vi "Dialog_TestGIV (SubVI).vi"() -> ()   [LabVIEW 2017]
uses:
  <vilib>/Waveform/WDTFileIO.llb/ Write Waveforms to File (1D).vi
panel:
  in  "Stop":bool
  in  "ExpClipboard":bool
  in  "UNDT_NOut":u8=1 caption="№ ПЭП подкл. к ГИВ" min=1 max=8 step=1
  out "Horizontal Fill Indicator":dbl(slide)=1.0 scale=0.0..1.0
  in  "Tab Control 2":enum32{"Osc", "Table", "Parameters"}(tab)
  out "OscPulse":waveform(dbl)[](graph)=[{"t0"=timestamp(0 s since 1904-01-01), "dt"=2.000000026702864e-10, "Y"=array[2502 elements]}, {"t0"=timestamp(0 s since 1904-01-01), "dt"=2.000000026702864e-10, "Y"=array[2502 elements]}, {"t0"=timestamp(0 s since 1904-01-01), "dt"=2.000000026702864e-10, "Y"=array[2502 elements]}, {"t0"=timestamp(0 s since 1904-01-01), "dt"=2.000000026702864e-10, "Y"=array[2502 elements]}, {"t0"=timestamp(0 s since 1904-01-01), "dt"=2.000000026702864e-10, "Y"=array[2502 elements]}, {"t0"=timestamp(0 s since 1904-01-01), "dt"=2.000000026702864e-10, "Y"=array[2502 elements]}, {"t0"=timestamp(0 s since 1904-01-01), "dt"=4.000000053405728e-10, "Y"=array[5002 elements]}, {"t0"=timestamp(0 s since 1904-01-01), "dt"=4.000000053405728e-10, "Y"=array[5002 elements]}, {"t0"=timestamp(0 s since 1904-01-01), "dt"=4.000000053405728e-10, "Y"=array[5002 elements]}, {"t0"=timestamp(0 s since 1904-01-01), "dt"=4.000000053405728e-10, "Y"=array[5002 elements]}, {"t0"=timestamp(0 s since 1904-01-01), "dt"=2.000000026702864e-10, "Y"=array[2502 elements]}, {"t0"=timestamp(0 s since 1904-01-01), "dt"=2.000000026702864e-10, "Y"=array[2502 elements]}, {"t0"=timestamp(0 s since 1904-01-01), "dt"=2.000000026702864e-10, "Y"=array[2502 elements]}, {"t0"=timestamp(0 s since 1904-01-01), "dt"=2.000000026702864e-10, "Y"=array[2502 elements]}, {"t0"=timestamp(0 s since 1904-01-01), "dt"=2.000000026702864e-10, "Y"=array[2502 elements]}, {"t0"=timestamp(0 s since 1904-01-01), "dt"=2.000000026702864e-10, "Y"=array[2502 elements]}, {"t0"=timestamp(0 s since 1904-01-01), "dt"=4.000000053405728e-10, "Y"=array[5002 elements]}, {"t0"=timestamp(0 s since 1904-01-01), "dt"=4.000000053405728e-10, "Y"=array[5002 elements]}, {"t0"=timestamp(0 s since 1904-01-01), "dt"=4.000000053405728e-10, "Y"=array[5002 elements]}, {"t0"=timestamp(0 s since 1904-01-01), "dt"=4.000000053405728e-10, "Y"=array[5002 elements]}, {"t0"=timestamp(0 s since 1904-01-01), "dt"=2.000000026702864e-10, "Y"=array[2502 elements]}, {"t0"=timestamp(0 s since 1904-01-01), "dt"=2.000000026702864e-10, "Y"=array[2502 elements]}, {"t0"=timestamp(0 s since 1904-01-01), "dt"=2.000000026702864e-10, "Y"=array[2502 elements]}, {"t0"=timestamp(0 s since 1904-01-01), "dt"=2.000000026702864e-10, "Y"=array[2502 elements]}, {"t0"=timestamp(0 s since 1904-01-01), "dt"=2.000000026702864e-10, "Y"=array[2502 elements]}, {"t0"=timestamp(0 s since 1904-01-01), "dt"=2.000000026702864e-10, "Y"=array[2502 elements]}, {"t0"=timestamp(0 s since 1904-01-01), "dt"=4.000000053405728e-10, "Y"=array[5002 elements]}, {"t0"=timestamp(0 s since 1904-01-01), "dt"=4.000000053405728e-10, "Y"=array[5002 elements]}, {"t0"=timestamp(0 s since 1904-01-01), "dt"=4.000000053405728e-10, "Y"=array[5002 elements]}, {"t0"=timestamp(0 s since 1904-01-01), "dt"=4.000000053405728e-10, "Y"=array[5002 elements]}, {"t0"=timestamp(0 s since 1904-01-01), "dt"=2.000000026702864e-10, "Y"=array[2502 elements]}, {"t0"=timestamp(0 s since 1904-01-01), "dt"=2.000000026702864e-10, "Y"=array[2502 elements]}, {"t0"=timestamp(0 s since 1904-01-01), "dt"=2.000000026702864e-10, "Y"=array[2502 elements]}, {"t0"=timestamp(0 s since 1904-01-01), "dt"=2.000000026702864e-10, "Y"=array[2502 elements]}, {"t0"=timestamp(0 s since 1904-01-01), "dt"=2.000000026702864e-10, "Y"=array[2502 elements]}, {"t0"=timestamp(0 s since 1904-01-01), "dt"=2.000000026702864e-10, "Y"=array[2502 elements]}, {"t0"=timestamp(0 s since 1904-01-01), "dt"=4.000000053405728e-10, "Y"=array[5002 elements]}, {"t0"=timestamp(0 s since 1904-01-01), "dt"=4.000000053405728e-10, "Y"=array[5002 elements]}, {"t0"=timestamp(0 s since 1904-01-01), "dt"=4.000000053405728e-10, "Y"=array[5002 elements]}, {"t0"=timestamp(0 s since 1904-01-01), "dt"=4.000000053405728e-10, "Y"=array[5002 elements]}, {"t0"=timestamp(0 s since 1904-01-01), "dt"=2.000000026702864e-10, "Y"=array[2502 elements]}, {"t0"=timestamp(0 s since 1904-01-01), "dt"=2.000000026702864e-10, "Y"=array[2502 elements]}, {"t0"=timestamp(0 s since 1904-01-01), "dt"=2.000000026702864e-10, "Y"=array[2502 elements]}, {"t0"=timestamp(0 s since 1904-01-01), "dt"=2.000000026702864e-10, "Y"=array[2502 elements]}, {"t0"=timestamp(0 s since 1904-01-01), "dt"=2.000000026702864e-10, "Y"=array[2502 elements]}, {"t0"=timestamp(0 s since 1904-01-01), "dt"=2.000000026702864e-10, "Y"=array[2502 elements]}, {"t0"=timestamp(0 s since 1904-01-01), "dt"=4.000000053405728e-10, "Y"=array[5002 elements]}, {"t0"=timestamp(0 s since 1904-01-01), "dt"=4.000000053405728e-10, "Y"=array[5002 elements]}, {"t0"=timestamp(0 s since 1904-01-01), "dt"=4.000000053405728e-10, "Y"=array[5002 elements]}, {"t0"=timestamp(0 s since 1904-01-01), "dt"=4.000000053405728e-10, "Y"=array[5002 elements]}, {"t0"=timestamp(0 s since 1904-01-01), "dt"=2.000000026702864e-10, "Y"=array[2502 elements]}, {"t0"=timestamp(0 s since 1904-01-01), "dt"=2.000000026702864e-10, "Y"=array[2502 elements]}, {"t0"=timestamp(0 s since 1904-01-01), "dt"=2.000000026702864e-10, "Y"=array[2502 elements]}, {"t0"=timestamp(0 s since 1904-01-01), "dt"=2.000000026702864e-10, "Y"=array[2502 elements]}, {"t0"=timestamp(0 s since 1904-01-01), "dt"=2.000000026702864e-10, "Y"=array[2502 elements]}, {"t0"=timestamp(0 s since 1904-01-01), "dt"=2.000000026702864e-10, "Y"=array[2502 elements]}, {"t0"=timestamp(0 s since 1904-01-01), "dt"=4.000000053405728e-10, "Y"=array[5002 elements]}, {"t0"=timestamp(0 s since 1904-01-01), "dt"=4.000000053405728e-10, "Y"=array[5002 elements]}, {"t0"=timestamp(0 s since 1904-01-01), "dt"=4.000000053405728e-10, "Y"=array[5002 elements]}, {"t0"=timestamp(0 s since 1904-01-01), "dt"=4.000000053405728e-10, "Y"=array[5002 elements]}, {"t0"=timestamp(0 s since 1904-01-01), "dt"=2.000000026702864e-10, "Y"=array[2502 elements]}, {"t0"=timestamp(0 s since 1904-01-01), "dt"=2.000000026702864e-10, "Y"=array[2502 elements]}, {"t0"=timestamp(0 s since 1904-01-01), "dt"=2.000000026702864e-10, "Y"=array[2502 elements]}, {"t0"=timestamp(0 s since 1904-01-01), "dt"=2.000000026702864e-10, "Y"=array[2502 elements]}, {"t0"=timestamp(0 s since 1904-01-01), "dt"=2.000000026702864e-10, "Y"=array[2502 elements]}, {"t0"=timestamp(0 s since 1904-01-01), "dt"=2.000000026702864e-10, "Y"=array[2502 elements]}, {"t0"=timestamp(0 s since 1904-01-01), "dt"=4.000000053405728e-10, "Y"=array[5002 elements]}, {"t0"=timestamp(0 s since 1904-01-01), "dt"=4.000000053405728e-10, "Y"=array[5002 elements]}, {"t0"=timestamp(0 s since 1904-01-01), "dt"=4.000000053405728e-10, "Y"=array[5002 elements]}, {"t0"=timestamp(0 s since 1904-01-01), "dt"=4.000000053405728e-10, "Y"=array[5002 elements]}, {"t0"=timestamp(0 s since 1904-01-01), "dt"=2.000000026702864e-10, "Y"=array[2502 elements]}, {"t0"=timestamp(0 s since 1904-01-01), "dt"=2.000000026702864e-10, "Y"=array[2502 elements]}, {"t0"=timestamp(0 s since 1904-01-01), "dt"=2.000000026702864e-10, "Y"=array[2502 elements]}, {"t0"=timestamp(0 s since 1904-01-01), "dt"=2.000000026702864e-10, "Y"=array[2502 elements]}, {"t0"=timestamp(0 s since 1904-01-01), "dt"=2.000000026702864e-10, "Y"=array[2502 elements]}, {"t0"=timestamp(0 s since 1904-01-01), "dt"=2.000000026702864e-10, "Y"=array[2502 elements]}, {"t0"=timestamp(0 s since 1904-01-01), "dt"=4.000000053405728e-10, "Y"=array[5002 elements]}, {"t0"=timestamp(0 s since 1904-01-01), "dt"=4.000000053405728e-10, "Y"=array[5002 elements]}, {"t0"=timestamp(0 s since 1904-01-01), "dt"=4.000000053405728e-10, "Y"=array[5002 elements]}, {"t0"=timestamp(0 s since 1904-01-01), "dt"=4.000000053405728e-10, "Y"=array[5002 elements]}, {"t0"=timestamp(0 s since 1904-01-01), "dt"=2.000000026702864e-10, "Y"=array[2502 elements]}, {"t0"=timestamp(0 s since 1904-01-01), "dt"=2.000000026702864e-10, "Y"=array[2502 elements]}, {"t0"=timestamp(0 s since 1904-01-01), "dt"=2.000000026702864e-10, "Y"=array[2502 elements]}, {"t0"=timestamp(0 s since 1904-01-01), "dt"=2.000000026702864e-10, "Y"=array[2502 elements]}, {"t0"=timestamp(0 s since 1904-01-01), "dt"=2.000000026702864e-10, "Y"=array[2502 elements]}, {"t0"=timestamp(0 s since 1904-01-01), "dt"=2.000000026702864e-10, "Y"=array[2502 elements]}, {"t0"=timestamp(0 s since 1904-01-01), "dt"=4.000000053405728e-10, "Y"=array[5002 elements]}, {"t0"=timestamp(0 s since 1904-01-01), "dt"=4.000000053405728e-10, "Y"=array[5002 elements]}, {"t0"=timestamp(0 s since 1904-01-01), "dt"=4.000000053405728e-10, "Y"=array[5002 elements]}, {"t0"=timestamp(0 s since 1904-01-01), "dt"=4.000000053405728e-10, "Y"=array[5002 elements]}, {"t0"=timestamp(0 s since 1904-01-01), "dt"=2.000000026702864e-10, "Y"=array[2502 elements]}, {"t0"=timestamp(0 s since 1904-01-01), "dt"=2.000000026702864e-10, "Y"=array[2502 elements]}, {"t0"=timestamp(0 s since 1904-01-01), "dt"=2.000000026702864e-10, "Y"=array[2502 elements]}, {"t0"=timestamp(0 s since 1904-01-01), "dt"=2.000000026702864e-10, "Y"=array[2502 elements]}, {"t0"=timestamp(0 s since 1904-01-01), "dt"=2.000000026702864e-10, "Y"=array[2502 elements]}, {"t0"=timestamp(0 s since 1904-01-01), "dt"=2.000000026702864e-10, "Y"=array[2502 elements]}, {"t0"=timestamp(0 s since 1904-01-01), "dt"=4.000000053405728e-10, "Y"=array[5002 elements]}, {"t0"=timestamp(0 s since 1904-01-01), "dt"=4.000000053405728e-10, "Y"=array[5002 elements]}, {"t0"=timestamp(0 s since 1904-01-01), "dt"=4.000000053405728e-10, "Y"=array[5002 elements]}, {"t0"=timestamp(0 s since 1904-01-01), "dt"=4.000000053405728e-10, "Y"=array[5002 elements]}]
  out "2D Array":dbl[][][](array[numeric])=[[[19.1375, 7.541862500000001e-08, 21.759999999999998, 6.929262500000001e-08], [19.315, 1.0552737500000001e-07, 19.83, 1.0297399999999999e-07], [20.1375, 2.0163137500000002e-07, 20.458750000000002, 1.99900625e-07], [19.9925, 3.999428749999999e-07, 20.286249999999995, 3.9827225e-07], [19.90625, 9.973029999999998e-07, 20.16, 9.9602075e-07]], [[40.683749999999996, 6.506337499999999e-08, 41.54875, 6.380575e-08], [41.442499999999995, 1.00427875e-07, 42.04875, 9.877425000000002e-08], [42.38999999999999, 1.9803800000000004e-07, 43.13999999999999, 1.9611924999999996e-07], [41.871249999999996, 3.9689725000000004e-07, 42.69250000000001, 3.948975e-07], [41.72, 9.93895e-07, 42.387499999999996, 9.927427500000001e-07]], [[60.49999999999999, 6.178550000000001e-08, 61.18999999999999, 6.068925e-08], [61.77374999999999, 1.0110387500000001e-07, 61.96499999999999, 9.946074999999999e-08], [62.886250000000004, 1.9951899999999997e-07, 63.1925, 1.9868749999999997e-07], [62.118750000000006, 3.9824899999999993e-07, 62.31875, 3.974105e-07], [61.62375, 9.95079e-07, 61.88250000000001, 9.9540575e-07]], [[79.85625, 6.04025e-08, 80.10000000000001, 5.873075e-08], [80.88000000000001, 9.995824999999998e-08, 81.3325, 9.767012499999999e-08], [82.7375, 1.9920325e-07, 82.665, 1.9787574999999998e-07], [81.47375, 4.0271224999999994e-07, 81.81374999999998, 4.01481875e-07], [81.02375, 9.99599125e-07, 81.225, 9.99024e-07]], [[99.955, 5.887400000000001e-08, 100.39000000000001, 5.733025e-08], [101.7275, 9.953974999999998e-08, 101.7075, 9.80625e-08], [103.40124999999999, 1.9899150000000003e-07, 103.45875000000001, 1.97883125e-07], [101.98750000000001, 4.0150525e-07, 102.07749999999999, 3.9996950000000004e-07], [101.25750000000001, 9.98323625e-07, 101.39874999999999, 9.9785925e-07]], [[119.02000000000002, 5.7773250000000004e-08, 118.85625, 5.623987499999999e-08], [120.69125, 9.8349125e-08, 120.745, 9.7001e-08], [123.22125000000001, 1.9811375000000002e-07, 122.86, 1.9654525e-07], [121.51, 4.0022249999999993e-07, 121.30624999999998, 3.99223875e-07], [120.30749999999998, 9.97211e-07, 120.28249999999998, 9.969812500000001e-07]], [[138.775, 5.6684000000000007e-08, 140.07000000000002, 5.5186499999999996e-08], [141.6875, 9.952662500000002e-08, 143.17875, 9.765412500000001e-08], [144.20625, 2.01772125e-07, 144.8325, 2.0063175000000004e-07], [142.0575, 4.005486249999999e-07, 142.785, 3.9960600000000006e-07], [141.14499999999998, 9.97314e-07, 141.76500000000001, 9.975241250000001e-07]], [[156.16250000000002, 5.5836750000000005e-08, 156.8375, 5.44745e-08], [159.85, 9.856150000000002e-08, 160.82500000000002, 9.733474999999998e-08], [161.9, 2.0106575e-07, 162.4, 2.0012125e-07], [159.67499999999998, 3.996415e-07, 160.55, 3.99016e-07], [159.0, 9.96793125e-07, 159.6, 9.968689999999997e-07]], [[177.67499999999998, 5.662325e-08, 179.17499999999998, 5.478087499999999e-08], [180.425, 9.806825000000001e-08, 181.63750000000002, 9.676424999999999e-08], [183.3125, 2.0135924999999998e-07, 183.79999999999998, 2.0038999999999998e-07], [179.96250000000003, 4.000740000000001e-07, 181.125, 3.9910099999999994e-07], [179.25, 9.9724875e-07, 180.20000000000002, 9.967589999999999e-07]], [[197.17499999999998, 5.6210500000000006e-08, 198.3, 5.4171e-08], [200.7875, 1.0082874999999998e-07, 201.91250000000002, 9.978087499999998e-08], [203.6125, 2.0081774999999999e-07, 204.0, 1.9978725e-07], [200.81250000000003, 3.9950762499999997e-07, 201.41250000000002, 3.9875574999999994e-07], [199.525, 9.964351250000002e-07, 200.0375, 9.96336e-07]]] format="%_4g"
  out "Mean":dbl[][](array[numeric])=[[19.1375, 7.541862500000001e-08, 21.759999999999998, 6.929262500000001e-08], [19.315, 1.0552737500000001e-07, 19.83, 1.0297399999999999e-07], [20.1375, 2.0163137500000002e-07, 20.458750000000002, 1.99900625e-07], [19.9925, 3.999428749999999e-07, 20.286249999999995, 3.9827225e-07], [19.90625, 9.973029999999998e-07, 20.16, 9.9602075e-07], [40.683749999999996, 6.506337499999999e-08, 41.54875, 6.380575e-08], [41.442499999999995, 1.00427875e-07, 42.04875, 9.877425000000002e-08], [42.38999999999999, 1.9803800000000004e-07, 43.13999999999999, 1.9611924999999996e-07], [41.871249999999996, 3.9689725000000004e-07, 42.69250000000001, 3.948975e-07], [41.72, 9.93895e-07, 42.387499999999996, 9.927427500000001e-07], [60.49999999999999, 6.178550000000001e-08, 61.18999999999999, 6.068925e-08], [61.77374999999999, 1.0110387500000001e-07, 61.96499999999999, 9.946074999999999e-08], [62.886250000000004, 1.9951899999999997e-07, 63.1925, 1.9868749999999997e-07], [62.118750000000006, 3.9824899999999993e-07, 62.31875, 3.974105e-07], [61.62375, 9.95079e-07, 61.88250000000001, 9.9540575e-07], [79.85625, 6.04025e-08, 80.10000000000001, 5.873075e-08], [80.88000000000001, 9.995824999999998e-08, 81.3325, 9.767012499999999e-08], [82.7375, 1.9920325e-07, 82.665, 1.9787574999999998e-07], [81.47375, 4.0271224999999994e-07, 81.81374999999998, 4.01481875e-07], [81.02375, 9.99599125e-07, 81.225, 9.99024e-07], [99.955, 5.887400000000001e-08, 100.39000000000001, 5.733025e-08], [101.7275, 9.953974999999998e-08, 101.7075, 9.80625e-08], [103.40124999999999, 1.9899150000000003e-07, 103.45875000000001, 1.97883125e-07], [101.98750000000001, 4.0150525e-07, 102.07749999999999, 3.9996950000000004e-07], [101.25750000000001, 9.98323625e-07, 101.39874999999999, 9.9785925e-07], [119.02000000000002, 5.7773250000000004e-08, 118.85625, 5.623987499999999e-08], [120.69125, 9.8349125e-08, 120.745, 9.7001e-08], [123.22125000000001, 1.9811375000000002e-07, 122.86, 1.9654525e-07], [121.51, 4.0022249999999993e-07, 121.30624999999998, 3.99223875e-07], [120.30749999999998, 9.97211e-07, 120.28249999999998, 9.969812500000001e-07], [138.775, 5.6684000000000007e-08, 140.07000000000002, 5.5186499999999996e-08], [141.6875, 9.952662500000002e-08, 143.17875, 9.765412500000001e-08], [144.20625, 2.01772125e-07, 144.8325, 2.0063175000000004e-07], [142.0575, 4.005486249999999e-07, 142.785, 3.9960600000000006e-07], [141.14499999999998, 9.97314e-07, 141.76500000000001, 9.975241250000001e-07], [156.16250000000002, 5.5836750000000005e-08, 156.8375, 5.44745e-08], [159.85, 9.856150000000002e-08, 160.82500000000002, 9.733474999999998e-08], [161.9, 2.0106575e-07, 162.4, 2.0012125e-07], [159.67499999999998, 3.996415e-07, 160.55, 3.99016e-07], [159.0, 9.96793125e-07, 159.6, 9.968689999999997e-07], [177.67499999999998, 5.662325e-08, 179.17499999999998, 5.478087499999999e-08], [180.425, 9.806825000000001e-08, 181.63750000000002, 9.676424999999999e-08], [183.3125, 2.0135924999999998e-07, 183.79999999999998, 2.0038999999999998e-07], [179.96250000000003, 4.000740000000001e-07, 181.125, 3.9910099999999994e-07], [179.25, 9.9724875e-07, 180.20000000000002, 9.967589999999999e-07], [197.17499999999998, 5.6210500000000006e-08, 198.3, 5.4171e-08], [200.7875, 1.0082874999999998e-07, 201.91250000000002, 9.978087499999998e-08], [203.6125, 2.0081774999999999e-07, 204.0, 1.9978725e-07], [200.81250000000003, 3.9950762499999997e-07, 201.41250000000002, 3.9875574999999994e-07], [199.525, 9.964351250000002e-07, 200.0375, 9.96336e-07]]
  in  "t имп":dbl[](array[numeric])=[0.05, 0.1, 0.35, 0.5, 0.7, 1.0] min=0.05 max=1.0 step=0.01 format="%.2g"
  in  "Амплитуда ГИВ":T1(array[ring])=[enum."20", enum."40", enum."60", enum."80", enum."100", enum."120", enum."140", enum."160", enum."180", enum."200"]
  in  "Osc":refnum<visa-resource-name>="TCPIP0::192.168.1.230::inst0::INSTR"
  in  "TestGIV":bool
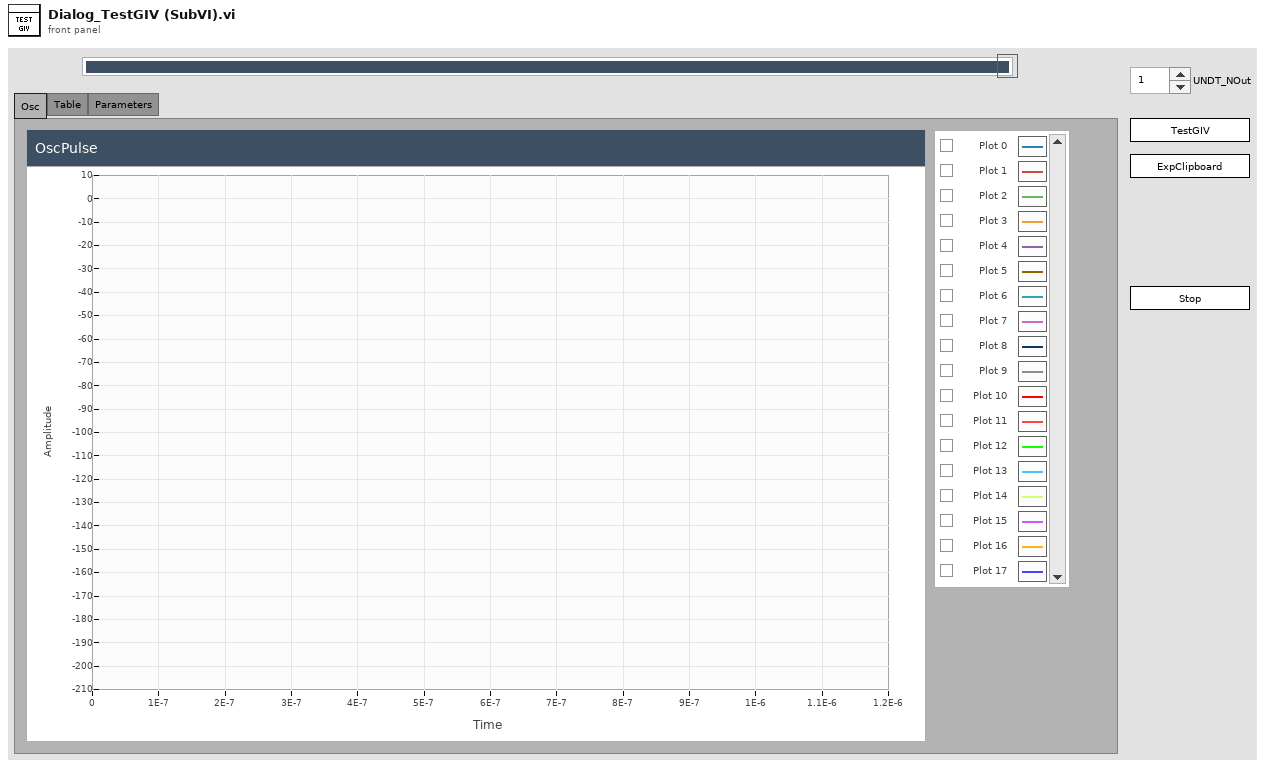
[diagram p1: front panel]
types:
  T1 = enum16{"20", "40", "60", "80", "100", "120", "140", "160", "180", "200"}[]
  T2 = cluster{"Vertical Range":dbl, "Channel":u16, "Vertical Coupling":u16, "Vertical Offset":dbl, "Probe Attenuation":dbl, "Bandwidth":u16, "Enable Channel":bool}[]
  T3 = cluster{"Maximum Sample Points":i32, "Timebase":dbl, "Position":dbl}
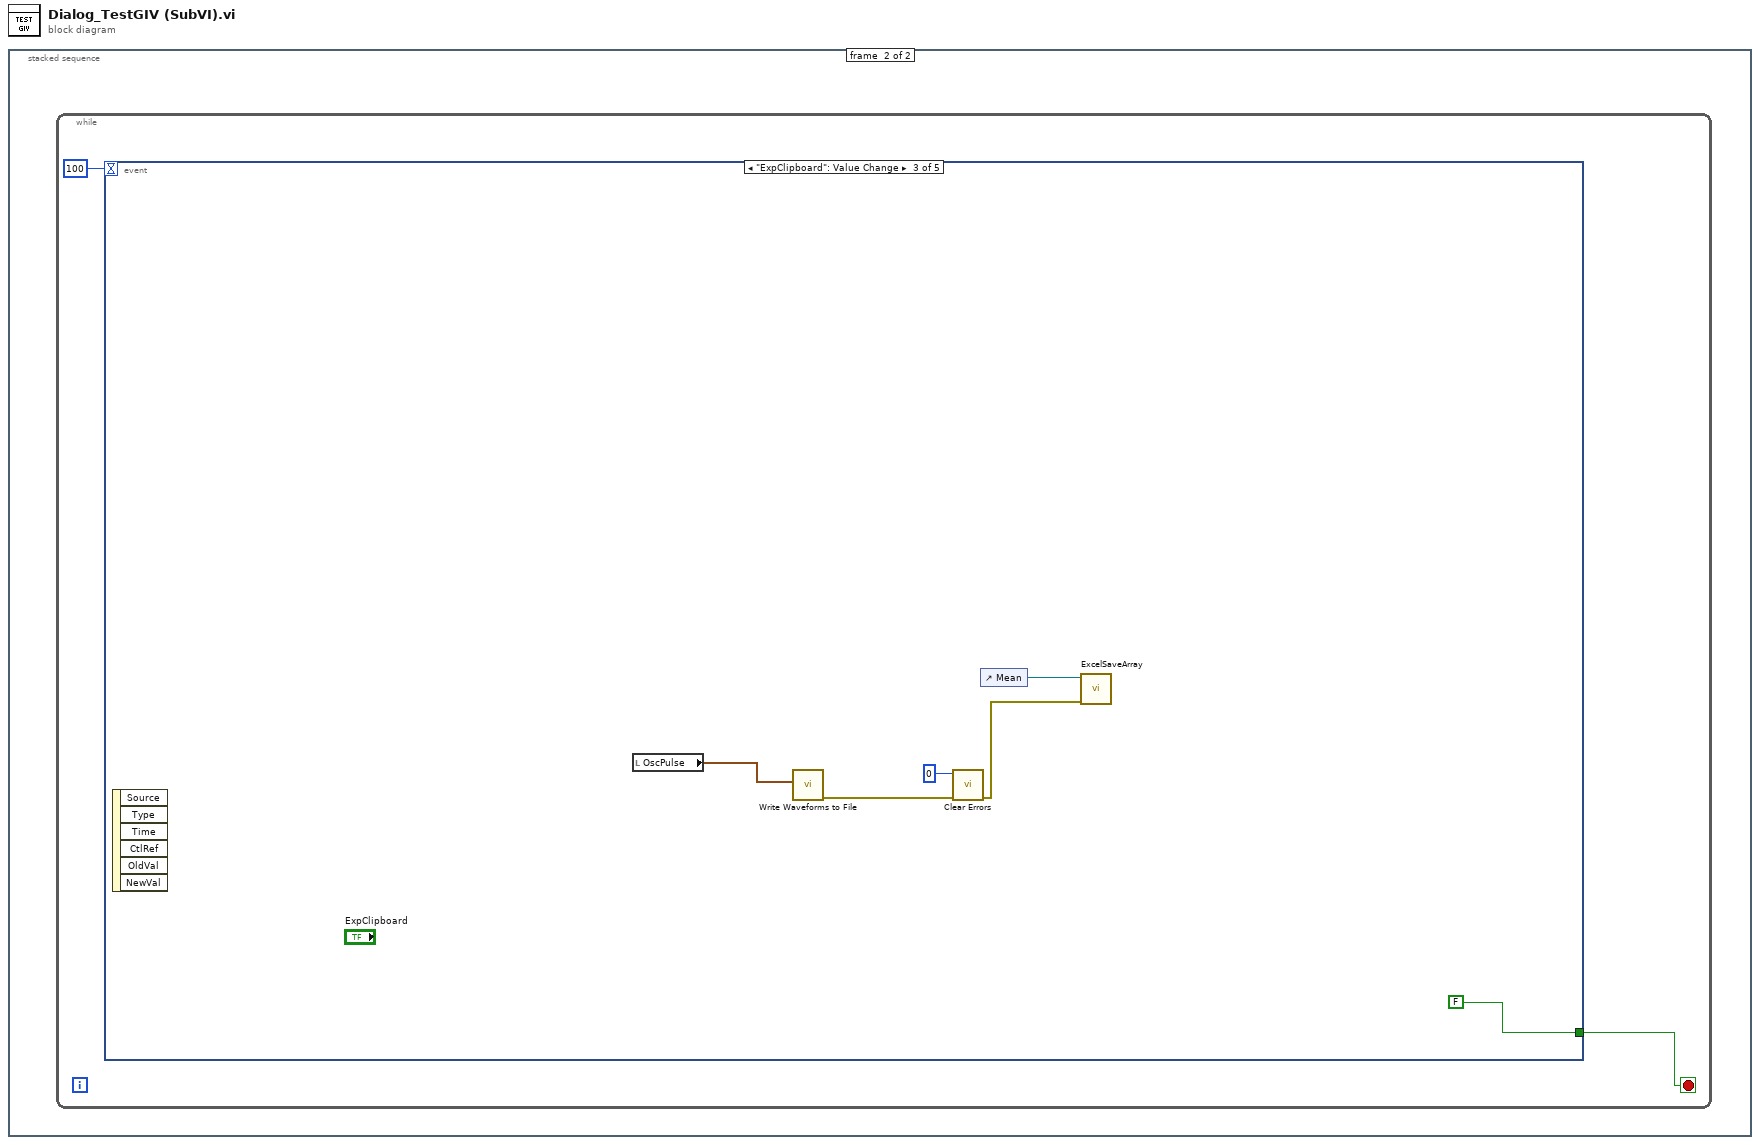
[diagram p0: block diagram]
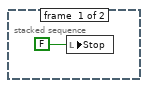
[diagram p2: hidden frame]
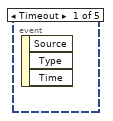
[diagram p3: hidden frame]
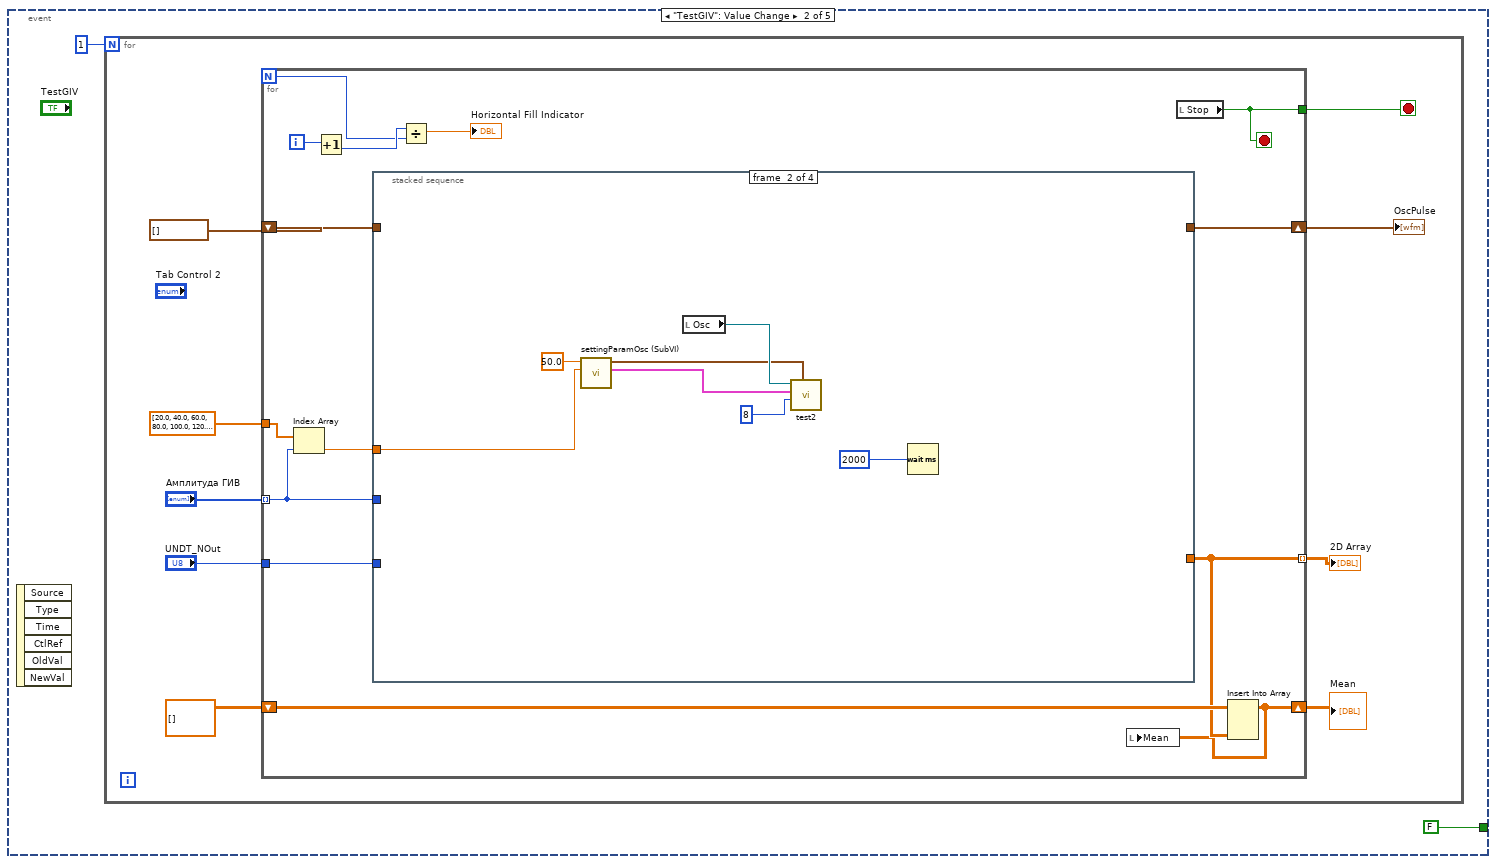
[diagram p4: hidden frame]
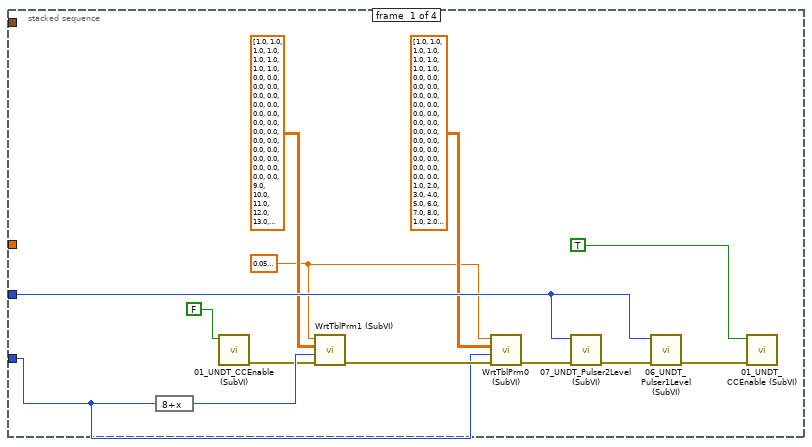
[diagram p5: hidden frame]
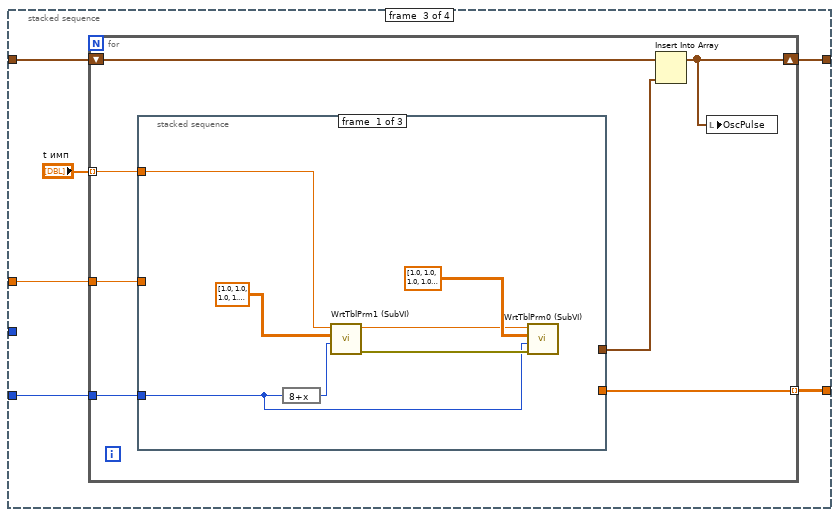
[diagram p6: hidden frame]
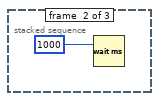
[diagram p7: hidden frame]
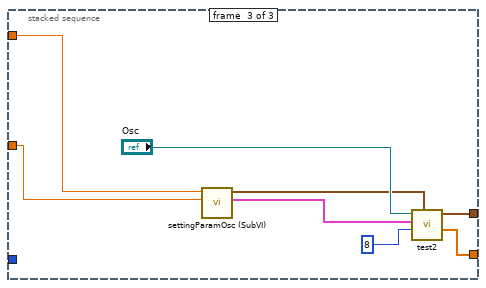
[diagram p8: hidden frame]
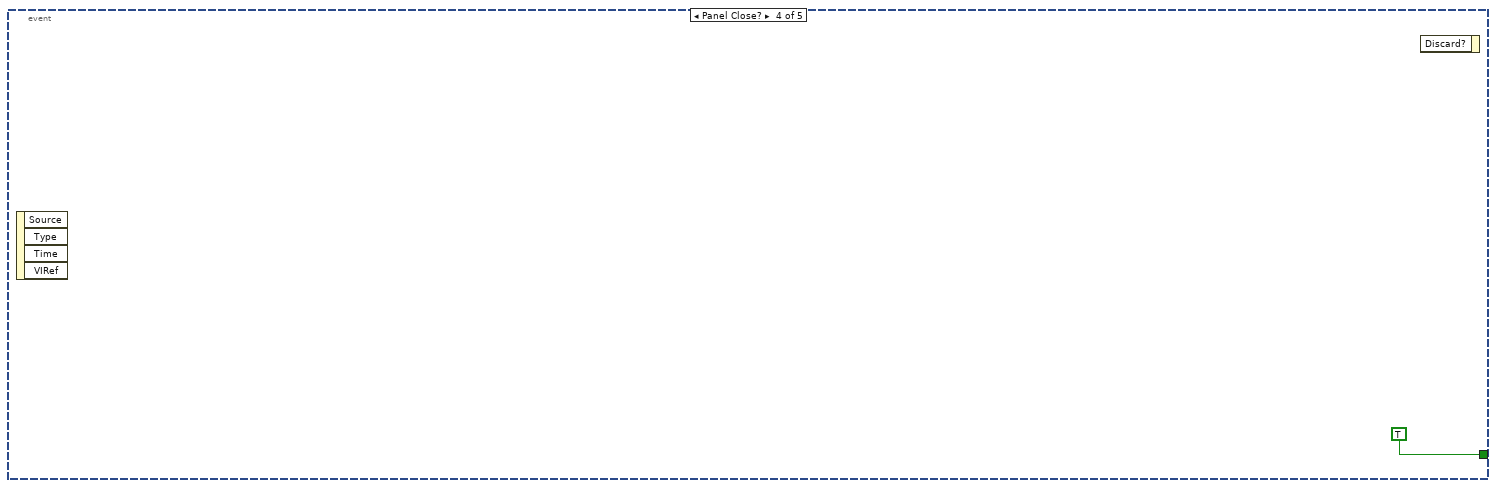
[diagram p10: hidden frame]
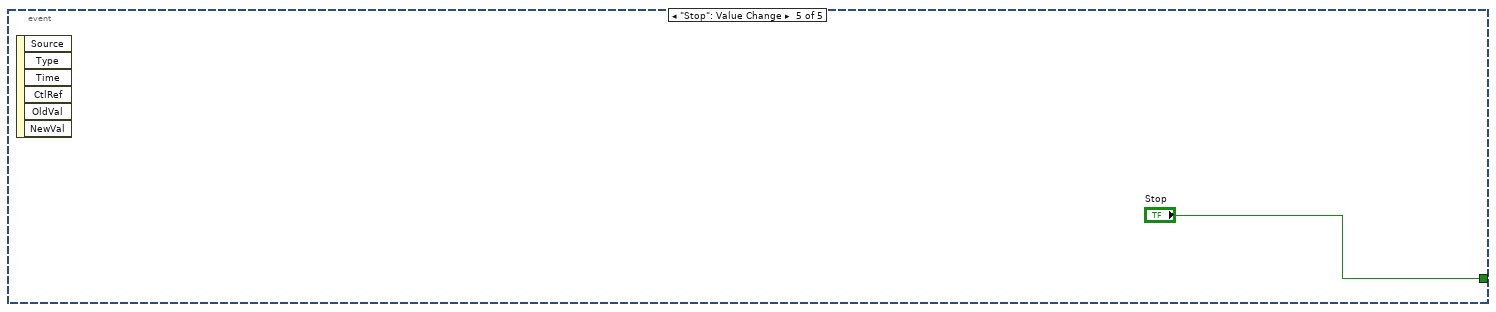
[diagram p11: hidden frame]
diagram:
  n1 = stacked-sequence {
    frame #0 {
      n2 = local write "Stop"(FALSE ("Stop")) -> ()
    }
    frame #1 {
      n3 = while {
        stop <- w2 stop-if-true
        n4 = event shown="[2] \"ExpClipboard\": Value Change" {
          selector: _ -> [_ _ _ _ _]
          dyn-events: _ -> [_ _ _ _ _]
          timeout: 100 -> [_ _ _ _ _]
          tunnel: [_ FALSE FALSE TRUE "Stop"] -> w2
          event Timeout {
            n5 = event-data() -> ()  [unwired: 1 in, 3 out]
          }
          event "TestGIV": Value Change {
            n6 = event-data() -> ()  [unwired: 1 in, 6 out]
            n7 = for {
              N: 1 -> [_]
              stop <- w6 stop-if-true
              n8 = for {
                N -> [w16]
                tunnel: "Амплитуда ГИВ" -> [w25] mode=indexing
                tunnel: [w21] -> w13 mode=indexing
                shift-right: [w28] -> w11
                shift-left: waveform(dbl)[] [] ("Osc") -> [w27]
                tunnel: dbl[] [20.0, 40.0, 60.0, 80.0, 100.0, 120.0, 140.0, 160.0, 180.0, 200.0] -> [w26]
                tunnel: "UNDT_NOut" -> [w23]
                shift-right: [w20] -> w7
                shift-left: dbl[][] [] ("Mean") -> [w22]
                tunnel: [w15] -> w6
                i -> [w19]
                stop <- w15 stop-if-true
                n9 = Index Array(array=w26, index=w25) -> (element=w24:dbl)
                n10 = Increment(x=w19) -> (x+1=w17:i32)
                n11 = stacked-sequence {
                  tunnel: [_ _ w53 _] -> w21
                  tunnel: w25 -> [w41 _ _ _]
                  tunnel: [_ _ w52 _] -> w28
                  tunnel: w27 -> [_ _ w51 _]
                  tunnel: w24 -> [_ w48 w50 _]
                  tunnel: w23 -> [w34 _ w49 _]
                  frame #0 {
                    w38 = sgl 0.05 ("t имп")
                    n12 = expression code="8+x"(w34) -> (w35:u8)
                    n13 = call "01_UNDT_CCEnable (SubVI).vi"("UNDT_Start"=FALSE) -> ("error out"=w29:errorcluster)  [unwired: 9 in, 1 out]
                    n14 = call "WrtTblPrm1 (SubVI).vi"("error in"=w29, "Nout"=w35, "TblPrm1"=sgl[][] [[1.0, 1.0, 1.0, 1.0, 1.0, 1.0, 1.0, 1.0, 0.0, 0.0, 0.0, 0.0, 0.0, 0.0, 0.0, 0.0, 0.0, 0.0, 0.0, 0.0, 0.0, 0.0, 0.0, 0.0, 0.0, 0.0, 0.0, 0.0, 0.0, 0.0, 0.0, 0.0], [9.0, 10.0, 11.0, 12.0, 13.0, 14.0, 15.0, 16.0, 9.0, 10.0, 11.0, 12.0, 13.0, 14.0, 15.0, 16.0, 9.0, 10.0, 11.0, 12.0, 13.0, 14.0, 15.0, 16.0, 9.0, 10.0, 11.0, 12.0, 13.0, 14.0, 15.0, 16.0], [0.0, 0.0, 0.0, 0.0, 0.0, 0.0, 0.0, 0.0, 0.0, 0.0, 0.0, 0.0, 0.0, 0.0, 0.0, 0.0, 0.0, 0.0, 0.0, 0.0, 0.0, 0.0, 0.0, 0.0, 0.0, 0.0, 0.0, 0.0, 0.0, 0.0, 0.0, 0.0], [0.3, 1.0, 1.0, 1.0, 1.0, 1.0, 1.0, 1.0, 0.1, 0.1, 0.1, 0.1, 0.1, 0.1, 0.1, 0.1, 0.1, 0.1, 0.1, 0.1, 0.1, 0.1, 0.1, 0.1, 0.1, 0.1, 0.1, 0.1, 0.1, 0.1, 0.1, 0.1], [1.0, 1.0, 1.0, 1.0, 1.0, 1.0, 1.0, 1.0, 1.0, 1.0, 1.0, 1.0, 1.0, 1.0, 1.0, 1.0, 1.0, 1.0, 1.0, 1.0, 1.0, 1.0, 1.0, 1.0, 1.0, 1.0, 1.0, 1.0, 1.0, 1.0, 1.0, 1.0], [9.0, 10.0, 11.0, 12.0, 13.0, 14.0, 15.0, 16.0, 9.0, 10.0, 11.0, 12.0, 13.0, 14.0, 15.0, 16.0, 9.0, 10.0, 11.0, 12.0, 13.0, 14.0, 15.0, 16.0, 9.0, 10.0, 11.0, 12.0, 13.0, 14.0, 15.0, 16.0], [0.0, 0.0, 0.0, 0.0, 0.0, 0.0, 0.0, 0.0, 0.0, 0.0, 0.0, 0.0, 0.0, 0.0, 0.0, 0.0, 0.0, 0.0, 0.0, 0.0, 0.0, 0.0, 0.0, 0.0, 0.0, 0.0, 0.0, 0.0, 0.0, 0.0, 0.0, 0.0], [1.0, 20.0, 20.0, 20.0, 20.0, 20.0, 20.0, 20.0, 20.0, 20.0, 20.0, 20.0, 20.0, 20.0, 20.0, 20.0, 20.0, 20.0, 20.0, 20.0, 20.0, 20.0, 20.0, 20.0, 20.0, 20.0, 20.0, 20.0, 20.0, 20.0, 20.0, 20.0], [0.0, 0.0, 0.0, 0.0, 0.0, 0.0, 0.0, 0.0, 0.0, 0.0, 0.0, 0.0, 0.0, 0.0, 0.0, 0.0, 0.0, 0.0, 0.0, 0.0, 0.0, 0.0, 0.0, 0.0, 0.0, 0.0, 0.0, 0.0, 0.0, 0.0, 0.0, 0.0], [999.0, 999.0, 999.0, 999.0, 999.0, 999.0, 999.0, 999.0, 999.0, 999.0, 999.0, 999.0, 999.0, 999.0, 999.0, 999.0, 999.0, 999.0, 999.0, 999.0, 999.0, 999.0, 999.0, 999.0, 999.0, 999.0, 999.0, 999.0, 999.0, 999.0, 999.0, 999.0]], "t имп"=w38) -> ("error out"=w37:errorcluster)  [unwired: 7 in]
                    n15 = call "WrtTblPrm0 (SubVI).vi"("error in"=w37, "Nout"=w34, "TblPrm0"=sgl[][] [[1.0, 1.0, 1.0, 1.0, 1.0, 1.0, 1.0, 1.0, 0.0, 0.0, 0.0, 0.0, 0.0, 0.0, 0.0, 0.0, 0.0, 0.0, 0.0, 0.0, 0.0, 0.0, 0.0, 0.0, 0.0, 0.0, 0.0, 0.0, 0.0, 0.0, 0.0, 0.0], [1.0, 2.0, 3.0, 4.0, 5.0, 6.0, 7.0, 8.0, 1.0, 2.0, 3.0, 4.0, 5.0, 6.0, 7.0, 8.0, 1.0, 2.0, 3.0, 4.0, 5.0, 6.0, 7.0, 8.0, 1.0, 2.0, 3.0, 4.0, 5.0, 6.0, 7.0, 8.0], [0.0, 0.0, 0.0, 0.0, 0.0, 0.0, 0.0, 0.0, 0.0, 0.0, 0.0, 0.0, 0.0, 0.0, 0.0, 0.0, 0.0, 0.0, 0.0, 0.0, 0.0, 0.0, 0.0, 0.0, 0.0, 0.0, 0.0, 0.0, 0.0, 0.0, 0.0, 0.0], [0.3, 1.0, 1.0, 1.0, 1.0, 1.0, 0.4, 1.0, 0.1, 0.1, 0.1, 0.1, 0.1, 0.1, 0.1, 0.1, 0.1, 0.1, 0.1, 0.1, 0.1, 0.1, 0.1, 0.1, 0.1, 0.1, 0.1, 0.1, 0.1, 0.1, 0.1, 0.1], [1.0, 1.0, 1.0, 1.0, 1.0, 1.0, 1.0, 1.0, 1.0, 1.0, 1.0, 1.0, 1.0, 1.0, 1.0, 1.0, 1.0, 1.0, 1.0, 1.0, 1.0, 1.0, 1.0, 1.0, 1.0, 1.0, 1.0, 1.0, 1.0, 1.0, 1.0, 1.0], [1.0, 2.0, 3.0, 4.0, 5.0, 6.0, 7.0, 8.0, 1.0, 2.0, 3.0, 4.0, 5.0, 6.0, 7.0, 8.0, 1.0, 2.0, 3.0, 4.0, 5.0, 6.0, 7.0, 8.0, 1.0, 2.0, 3.0, 4.0, 5.0, 6.0, 7.0, 8.0], [0.0, 0.0, 0.0, 0.0, 0.0, 0.0, 0.0, 0.0, 0.0, 0.0, 0.0, 0.0, 0.0, 0.0, 0.0, 0.0, 0.0, 0.0, 0.0, 0.0, 0.0, 0.0, 0.0, 0.0, 0.0, 0.0, 0.0, 0.0, 0.0, 0.0, 0.0, 0.0], [1.0, 20.0, 20.0, 20.0, 20.0, 20.0, 20.0, 20.0, 20.0, 20.0, 20.0, 20.0, 20.0, 20.0, 20.0, 20.0, 20.0, 20.0, 20.0, 20.0, 20.0, 20.0, 20.0, 20.0, 20.0, 20.0, 20.0, 20.0, 20.0, 20.0, 20.0, 20.0], [0.0, 0.0, 0.0, 0.0, 0.0, 0.0, 0.0, 0.0, 0.0, 0.0, 0.0, 0.0, 0.0, 0.0, 0.0, 0.0, 0.0, 0.0, 0.0, 0.0, 0.0, 0.0, 0.0, 0.0, 0.0, 0.0, 0.0, 0.0, 0.0, 0.0, 0.0, 0.0], [999.0, 999.0, 999.0, 999.0, 999.0, 999.0, 999.0, 999.0, 999.0, 999.0, 999.0, 999.0, 999.0, 999.0, 999.0, 999.0, 999.0, 999.0, 999.0, 999.0, 999.0, 999.0, 999.0, 999.0, 999.0, 999.0, 999.0, 999.0, 999.0, 999.0, 999.0, 999.0]], "t имп"=w38) -> ("error out"=w31:errorcluster)  [unwired: 7 in]
                    n16 = call "07_UNDT_Pulser2Level (SubVI).vi"("error in"=w31, "UNDT_GIV2"=w41) -> ("error out"=w36:errorcluster)  [unwired: 9 in]
                    n17 = call "06_UNDT_Pulser1Level (SubVI).vi"("error in"=w36, "UNDT_GIV1"=w41) -> ("error out"=w30:errorcluster)  [unwired: 9 in]
                    n18 = call "01_UNDT_CCEnable (SubVI).vi"("error in"=w30, "UNDT_Start"=TRUE) -> ()  [unwired: 8 in, 2 out]
                  }
                  frame #1 {
                    n19 = call "settingParamOsc (SubVI).vi"("Volt"=w48, "UNDT_Pulse"=50.0) -> ("Array"=w45:T2, "Time"=w42:T3)  [unwired: 8 in]
                    n20 = local read "Osc"() -> (w46:refnum<visa-resource-name>)
                    n21 = call "test2.vi"("Time"=w42, "NAveraging"=8, "Channel config"=w45, "VISA resource name"=w46) -> ()  [unwired: 5 in, 3 out]
                    n22 = Wait (ms)(milliseconds to wait=u32 2000) -> ()  [unwired: 1 out]
                  }
                  frame #2 {
                    n23 = for {
                      tunnel: "t имп" -> [w61] mode=indexing
                      shift-right: [w57] -> w52
                      shift-left: w51 -> [w60]
                      tunnel: [w58] -> w53 mode=indexing
                      tunnel: w50 -> [w56]
                      tunnel: w49 -> [w55]
                      n24 = stacked-sequence {
                        tunnel: w61 -> [w65 _ w73]
                        tunnel: [_ _ w76] -> w59
                        tunnel: [_ _ w75] -> w58
                        tunnel: w56 -> [_ _ w74]
                        tunnel: w55 -> [w62 _ _]
                        frame #0 {
                          n25 = expression code="8+x"(w62) -> (w63:u8)
                          n26 = call "WrtTblPrm1 (SubVI).vi"("Nout"=w63, "TblPrm1"=sgl[][] [[1.0, 1.0, 1.0, 1.0, 1.0, 1.0, 1.0, 1.0, 0.0, 0.0, 0.0, 0.0, 0.0, 0.0, 0.0, 0.0, 0.0, 0.0, 0.0, 0.0, 0.0, 0.0, 0.0, 0.0, 0.0, 0.0, 0.0, 0.0, 0.0, 0.0, 0.0, 0.0], [16.0, 10.0, 11.0, 12.0, 13.0, 14.0, 15.0, 16.0, 9.0, 10.0, 11.0, 12.0, 13.0, 14.0, 15.0, 16.0, 9.0, 10.0, 11.0, 12.0, 13.0, 14.0, 15.0, 16.0, 9.0, 10.0, 11.0, 12.0, 13.0, 14.0, 15.0, 16.0], [0.0, 0.0, 0.0, 0.0, 0.0, 0.0, 0.0, 0.0, 0.0, 0.0, 0.0, 0.0, 0.0, 0.0, 0.0, 0.0, 0.0, 0.0, 0.0, 0.0, 0.0, 0.0, 0.0, 0.0, 0.0, 0.0, 0.0, 0.0, 0.0, 0.0, 0.0, 0.0], [0.3, 1.0, 1.0, 1.0, 1.0, 1.0, 1.0, 1.0, 0.1, 0.1, 0.1, 0.1, 0.1, 0.1, 0.1, 0.1, 0.1, 0.1, 0.1, 0.1, 0.1, 0.1, 0.1, 0.1, 0.1, 0.1, 0.1, 0.1, 0.1, 0.1, 0.1, 0.1], [1.0, 1.0, 1.0, 1.0, 1.0, 1.0, 1.0, 1.0, 1.0, 1.0, 1.0, 1.0, 1.0, 1.0, 1.0, 1.0, 1.0, 1.0, 1.0, 1.0, 1.0, 1.0, 1.0, 1.0, 1.0, 1.0, 1.0, 1.0, 1.0, 1.0, 1.0, 1.0], [9.0, 10.0, 11.0, 12.0, 13.0, 14.0, 15.0, 16.0, 9.0, 10.0, 11.0, 12.0, 13.0, 14.0, 15.0, 16.0, 9.0, 10.0, 11.0, 12.0, 13.0, 14.0, 15.0, 16.0, 9.0, 10.0, 11.0, 12.0, 13.0, 14.0, 15.0, 16.0], [0.0, 0.0, 0.0, 0.0, 0.0, 0.0, 0.0, 0.0, 0.0, 0.0, 0.0, 0.0, 0.0, 0.0, 0.0, 0.0, 0.0, 0.0, 0.0, 0.0, 0.0, 0.0, 0.0, 0.0, 0.0, 0.0, 0.0, 0.0, 0.0, 0.0, 0.0, 0.0], [20.0, 20.0, 20.0, 20.0, 20.0, 20.0, 20.0, 20.0, 20.0, 20.0, 20.0, 20.0, 20.0, 20.0, 20.0, 20.0, 20.0, 20.0, 20.0, 20.0, 20.0, 20.0, 20.0, 20.0, 20.0, 20.0, 20.0, 20.0, 20.0, 20.0, 20.0, 20.0], [0.0, 0.0, 0.0, 0.0, 0.0, 0.0, 0.0, 0.0, 0.0, 0.0, 0.0, 0.0, 0.0, 0.0, 0.0, 0.0, 0.0, 0.0, 0.0, 0.0, 0.0, 0.0, 0.0, 0.0, 0.0, 0.0, 0.0, 0.0, 0.0, 0.0, 0.0, 0.0], [999.0, 999.0, 999.0, 999.0, 999.0, 999.0, 999.0, 999.0, 999.0, 999.0, 999.0, 999.0, 999.0, 999.0, 999.0, 999.0, 999.0, 999.0, 999.0, 999.0, 999.0, 999.0, 999.0, 999.0, 999.0, 999.0, 999.0, 999.0, 999.0, 999.0, 999.0, 999.0]], "t имп"=w65) -> ("error out"=w64:errorcluster)  [unwired: 8 in]
                          n27 = call "WrtTblPrm0 (SubVI).vi"("error in"=w64, "Nout"=w62, "TblPrm0"=sgl[][] [[1.0, 1.0, 1.0, 1.0, 1.0, 1.0, 1.0, 1.0, 0.0, 0.0, 0.0, 0.0, 0.0, 0.0, 0.0, 0.0, 0.0, 0.0, 0.0, 0.0, 0.0, 0.0, 0.0, 0.0, 0.0, 0.0, 0.0, 0.0, 0.0, 0.0, 0.0, 0.0], [1.0, 2.0, 3.0, 4.0, 5.0, 6.0, 7.0, 8.0, 1.0, 2.0, 3.0, 4.0, 5.0, 6.0, 7.0, 8.0, 1.0, 2.0, 3.0, 4.0, 5.0, 6.0, 7.0, 8.0, 1.0, 2.0, 3.0, 4.0, 5.0, 6.0, 7.0, 8.0], [0.0, 0.0, 0.0, 0.0, 0.0, 0.0, 0.0, 0.0, 0.0, 0.0, 0.0, 0.0, 0.0, 0.0, 0.0, 0.0, 0.0, 0.0, 0.0, 0.0, 0.0, 0.0, 0.0, 0.0, 0.0, 0.0, 0.0, 0.0, 0.0, 0.0, 0.0, 0.0], [0.3, 1.0, 1.0, 1.0, 1.0, 1.0, 0.4, 1.0, 0.1, 0.1, 0.1, 0.1, 0.1, 0.1, 0.1, 0.1, 0.1, 0.1, 0.1, 0.1, 0.1, 0.1, 0.1, 0.1, 0.1, 0.1, 0.1, 0.1, 0.1, 0.1, 0.1, 0.1], [1.0, 1.0, 1.0, 1.0, 1.0, 1.0, 1.0, 1.0, 1.0, 1.0, 1.0, 1.0, 1.0, 1.0, 1.0, 1.0, 1.0, 1.0, 1.0, 1.0, 1.0, 1.0, 1.0, 1.0, 1.0, 1.0, 1.0, 1.0, 1.0, 1.0, 1.0, 1.0], [1.0, 2.0, 3.0, 4.0, 5.0, 6.0, 7.0, 8.0, 1.0, 2.0, 3.0, 4.0, 5.0, 6.0, 7.0, 8.0, 1.0, 2.0, 3.0, 4.0, 5.0, 6.0, 7.0, 8.0, 1.0, 2.0, 3.0, 4.0, 5.0, 6.0, 7.0, 8.0], [0.0, 0.0, 0.0, 0.0, 0.0, 0.0, 0.0, 0.0, 0.0, 0.0, 0.0, 0.0, 0.0, 0.0, 0.0, 0.0, 0.0, 0.0, 0.0, 0.0, 0.0, 0.0, 0.0, 0.0, 0.0, 0.0, 0.0, 0.0, 0.0, 0.0, 0.0, 0.0], [20.0, 20.0, 20.0, 20.0, 20.0, 20.0, 20.0, 20.0, 20.0, 20.0, 20.0, 20.0, 20.0, 20.0, 20.0, 20.0, 20.0, 20.0, 20.0, 20.0, 20.0, 20.0, 20.0, 20.0, 20.0, 20.0, 20.0, 20.0, 20.0, 20.0, 20.0, 20.0], [0.0, 0.0, 0.0, 0.0, 0.0, 0.0, 0.0, 0.0, 0.0, 0.0, 0.0, 0.0, 0.0, 0.0, 0.0, 0.0, 0.0, 0.0, 0.0, 0.0, 0.0, 0.0, 0.0, 0.0, 0.0, 0.0, 0.0, 0.0, 0.0, 0.0, 0.0, 0.0], [999.0, 999.0, 999.0, 999.0, 999.0, 999.0, 999.0, 999.0, 999.0, 999.0, 999.0, 999.0, 999.0, 999.0, 999.0, 999.0, 999.0, 999.0, 999.0, 999.0, 999.0, 999.0, 999.0, 999.0, 999.0, 999.0, 999.0, 999.0, 999.0, 999.0, 999.0, 999.0]], "t имп"=w65) -> ()  [unwired: 7 in, 1 out]
                        }
                        frame #1 {
                          n28 = Wait (ms)(milliseconds to wait=u32 1000) -> ()  [unwired: 1 out]
                        }
                        frame #2 {
                          n29 = call "settingParamOsc (SubVI).vi"("Volt"=w74, "UNDT_Pulse"=w73) -> ("Array"=w71:T2, "Time"=w69:T3)  [unwired: 8 in]
                          n30 = call "test2.vi"("Time"=w69, "NAveraging"=8, "Channel config"=w71, "VISA resource name"="Osc") -> ("Mean"=w75:dbl[], "Osc"=w76:waveform(dbl)[])  [unwired: 5 in, 1 out]
                        }
                      }
                      n31 = Insert Into Array(array=w60, new element=w59) -> (w57:waveform(dbl)[])  [unwired: 1 in]
                      n32 = local write "OscPulse"(w57) -> ()
                    }
                  }
                  frame #3 {
                  }
                }
                n33 = Divide(x=w17, y=w16) -> (x/y=→"Horizontal Fill Indicator":dbl)
                n34 = local read "Stop"() -> (w15:bool)
                n35 = Insert Into Array(array=w22, new element=w21) -> (w20:dbl[][])  [unwired: 2 in]
                n36 = local write "Mean"(w20) -> ()
              }
              "2D Array" <- w13
              "OscPulse" <- w11
              "Mean" <- w7
            }
          }
          event "ExpClipboard": Value Change {
            n37 = event-data() -> ()  [unwired: 1 in, 6 out]
            n38 = local read "OscPulse"() -> (w80:waveform(dbl)[])
            n39 = call-poly <vilib>:"Write Waveforms to File.vi"("waveform array"=w80) -> ("error out"=w79:errorcluster)  [unwired: 9 in, 1 out]
            n40 = call <vilib>:"Clear Errors.vi"("error in (no error)"=w79, "specific error code to clear (0: all)"=0) -> ("error out"=w77:errorcluster)  [unwired: 4 in, 1 out]
            n41 = control-ref of="Mean"() -> (w81:refnum<vi>)
            n42 = call "ExcelSaveArray.vi"("error in"=w77, "Mean"=w81) -> ()  [unwired: 9 in, 1 out]
          }
          event Panel Close? {
            n43 = event-data() -> ()  [unwired: 1 in, 4 out]
            n44 = event-data() -> ()  [unwired: 2 in, 1 out]
          }
          event "Stop": Value Change {
            n45 = event-data() -> ()  [unwired: 1 in, 6 out]
          }
        }
      }
    }
  }
